vi "create and send file.vi"(11 "list":cluster{"IP address":string, "output":string}[](array[cluster])) -> (0 "error out":errorcluster)   [LabVIEW 2020]
uses:
  <vilib>/Utility/config.llb/NI_LVConfig.lvlib
  <vilib>/WebDAVClient/NI_WebDAV.lvlib
  <vilib>/WebDAVClient/Advanced/Put File.vi
  <vilib>/Utility/config.llb/Write Key (String).vi
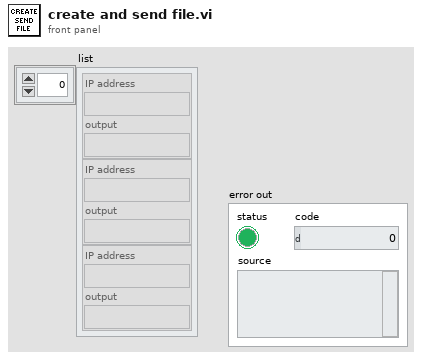
[diagram p1: front panel]
types:
  T1 = typedef "NI_LVConfig.lvlib/Config Data RefNum.ctl" = refnum<k1>
  T2 = typedef "NI_WebDAV.lvlib/SessionHandle.ctl" = refnum<k1>
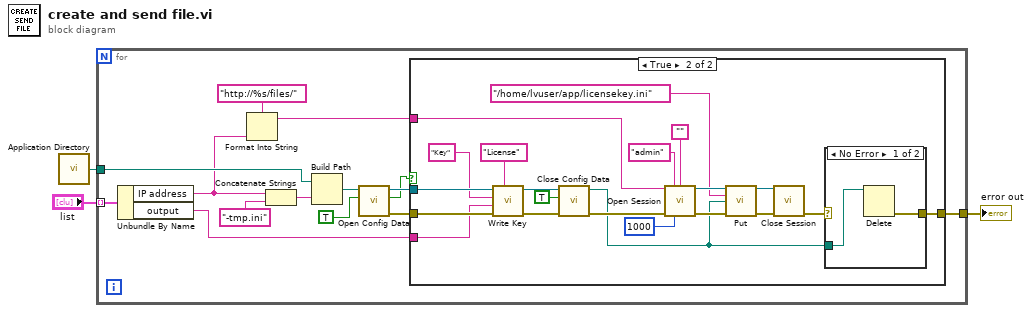
[diagram p0: block diagram]
diagram:
  n1 = call <vilib>:"Application Directory.vi"() -> ("Application Directory"=w3:path)
  n2 = for {
    tunnel: "list" -> [w14] mode=indexing
    tunnel: w3 -> [w13]
    tunnel: [w4] -> w1
    n3 = Unbundle By Name(w14) -> ("IP address"=w8:string, "output"=w10:string)
    n4 = Format Into String(format string="http://%s/files/" ("message queue name"), w8) -> (resulting string=w7:string)  [unwired: 2 in, 1 out]
    n5 = Concatenate Strings(w8, "-tmp.ini" ("message queue name")) -> (w12:string)
    n6 = Build Path(base path=w13, name or relative path=w12) -> (appended path=w15:path)
    n7 = call <vilib>:"Open Config Data.vi"("create file if necessary (T)"=TRUE ("write file if changed (T)"), "configuration file path"=w15) -> ("error out"=w17:errorcluster, "file created?"=w6:bool, "refnum"=w16:T1)  [unwired: 7 in]
    n8 = case shown="True" w6 {
      tunnel: w17 -> [_ w38]
      tunnel: w16 -> [_ w37]
      tunnel: w10 -> [_ w32]
      tunnel: w7 -> [_ w29]
      tunnel: [_ w18] -> w4
      frame False {
      }
      frame True {
        n9 = call-poly <vilib>:"Write Key.vi"("section"="License" ("message queue name"), "error in (no error)"=w38, "value"=w32, "key"="Key" ("message queue name"), "refnum"=w37) -> ("error out"=w35:errorcluster, "refnum out"=w36:T1)  [unwired: 4 in, 1 out]
        n10 = call <vilib>:"Close Config Data.vi"("error in (no error)"=w35, "write file if changed (T)"=TRUE, "refnum"=w36) -> ("error out"=w28:errorcluster, "file path"=w19:path)  [unwired: 7 in]
        n11 = call <vilib>:"Open Session.vi"("host uri prefix"=w29, "username"="admin" ("message queue name"), "password"="", "error in (no error)"=w28, "timeout ms"=1000) -> ("session handle out"=w26:T2, "error out"=w25:errorcluster)  [unwired: 9 in]
        n12 = call-poly <vilib>:"Put.vi"("session handle"=w26, "relative uri"="/home/lvuser/app/licensekey.ini" ("message queue name"), "local file path"=w19, "error in (no error)"=w25) -> ("session handle out"=w23:T2, "error out"=w22:errorcluster)  [unwired: 9 in, 1 out]
        n13 = call <vilib>:"Close Session.vi"("session handle"=w23, "error in (no error)"=w22) -> ("error out"=w20:errorcluster)  [unwired: 13 in]
        n14 = case shown="No Error" w20 {
          tunnel: w19 -> [w40 _]
          tunnel: [w39 _] -> w18
          frame No Error {
            n15 = Delete(path (use dialog)=w40) -> (error out=w39:errorcluster)  [unwired: 4 in, 2 out]
          }
          frame Error {
          }
        }
      }
    }
  }
  "error out" <- w1
